vi "Destroy.vi"(8 "Error In":errorcluster, 11 "reference in":refnum<class "CoconutMilkTea.lvclass">) -> (0 "Error Out":errorcluster, 3 "reference out":refnum<class "CoconutMilkTea.lvclass">)   [LabVIEW 2020, in "CoconutMilkTea.lvclass"]
uses:
  CoconutMilkTea.lvclass
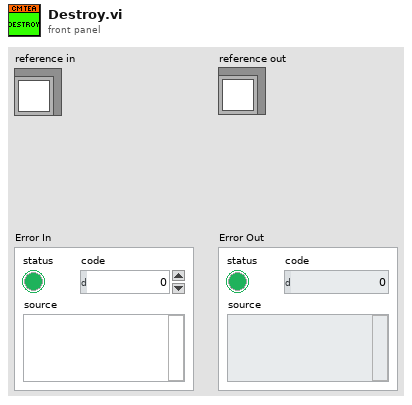
[diagram p1: front panel]
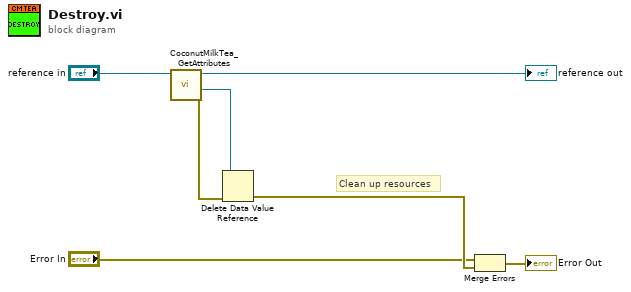
[diagram p0: block diagram]
diagram:
  # "Clean up resources"
  n1 = call "CoconutMilkTea_GetAttributes.vi"("reference in"="reference in") -> ("error out"=w4:errorcluster, "DataRef"=w3:refnum<data-value>, "reference out"=→"reference out":refnum<class "CoconutMilkTea.lvclass">)  [unwired: 7 in, 1 out]
  n2 = Delete Data Value Reference(data value reference=w3, error in=w4) -> (error out=w2:errorcluster)  [unwired: 1 out]
  n3 = Merge Errors("Error In", w2) -> (→"Error Out":errorcluster)
